vi "query field control mode.vi"(8 "error in (no error)":errorcluster, 11 "VISA session":refnum<visa-resource-name>) -> (0 "error out":errorcluster, 2 "Field Control Mode (0: Off)":u16(ring) items=["Off", "Closed Loop PI", "Manual"], 3 "dup VISA session":refnum<visa-resource-name>)   [LabVIEW 2017]
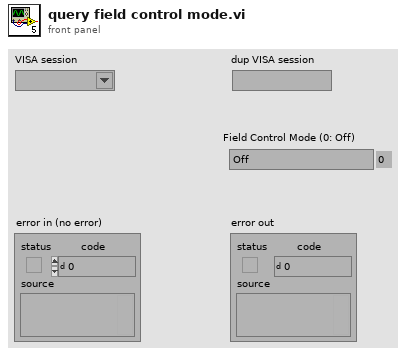
[diagram p1: front panel]
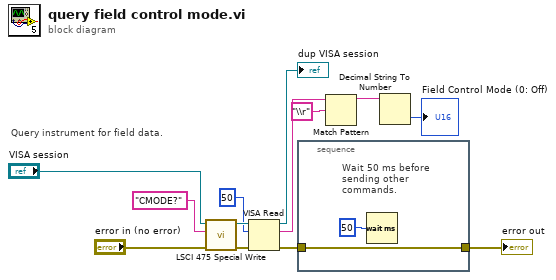
[diagram p0: block diagram]
diagram:
  # "Query instrument for field data."
  n1 = call "LSCI 475 Special Write.vi"("error in (no error)"="error in (no error)", "Write Buffer (\"\")"="CMODE?", "VISA session"="VISA session") -> ("error out"=w9:errorcluster, "dup VISA session"=w10:refnum<visa-resource-name>)  [unwired: 6 in, 1 out]
  n2 = VISA Read(VISA resource name=w10, byte count=u32 50, error in (no error)=w9) -> (VISA resource name out=→"dup VISA session":refnum<visa-resource-name>, read buffer=w2:string, error out=w6:errorcluster)  [unwired: 1 out]
  n3 = stacked-sequence {
    tunnel: w6 -> [w14]
    tunnel: [w14] -> w5
    frame #0 {
      # "Wait 50 ms before\nsending other\ncommands."
      n4 = Wait (ms)(milliseconds to wait=u32 50) -> ()  [unwired: 1 out]
    }
  }
  "error out" <- w5
  n5 = Match Pattern(string=w2, regular expression="\\r") -> (before substring=w1:string)  [unwired: 1 in, 3 out]
  n6 = Decimal String To Number(string=w1) -> (number=→"Field Control Mode (0: Off)":i32)  [unwired: 2 in, 1 out]
